vi "AdjustNames.vi"(8 "error in (no error)":errorcluster, 11 "Hardware In":T2 {"Logical Instrument"."Watchdog"."Interval (s)" min=1.0 max=360.0; "Logical Instrument"."Safety Trips"."Pmax Sink Time (s)" min=-1.0; "Logical Instrument"."Safety Trips"."Pmax Sink (W)" min=0.0 format="%#_7g"; "Logical Instrument"."Safety Trips"."Pmax Source Time (s)" min=-1.0; "Logical Instrument"."Safety Trips"."Pmax Source (W)" min=0.0 format="%#_7g"; "Logical Instrument"."Safety Trips"."Absolute Curr Peak" min=0.0; "Logical Instrument"."Safety Trips"."Imax Sink Time (s)" min=-1.0; "Logical Instrument"."Safety Trips"."Imax Sink (A)" min=0.0; "Logical Instrument"."Safety Trips"."Imax Source Time (s)" min=-1.0; "Logical Instrument"."Safety Trips"."Imax Source (A)" min=0.0; "Logical Instrument"."Safety Trips"."Absolute Volt Peak" min=0.0; "Logical Instrument"."Safety Trips"."Vmax Time (s)" min=-1.0; "Logical Instrument"."Safety Trips"."Vmax (V)" min=0.0; "Logical Instrument"."Safety Trips"."Vmin Time (s)" min=-1.0; "Logical Instrument"."Safety Trips"."Vmin (V)" min=0.0; "Logical Instrument"."Aperture (cycles)" min=1 max=64; "Logical Instrument"."FreqOut (Hz)" min=0.0 max=100.0; "Logical Instrument"."Slew Rates"."Phase Angle Min (Deg/s)" min=0.0; "Logical Instrument"."Slew Rates"."Phase Angle Max (Deg/s)" min=0.0; "Logical Instrument"."Slew Rates"."Freq Min (Hz/s)" min=0.0; "Logical Instrument"."Slew Rates"."Freq Max (Hz/s)" min=0.0; "Logical Instrument"."Slew Rates"."Pmax (W/s)" min=0.0; "Logical Instrument"."Slew Rates"."Pmin (W/s)" min=0.0; "Logical Instrument"."Slew Rates"."Imax (A/s)" min=0.0; "Logical Instrument"."Slew Rates"."Vmax (V/s)" min=0.0; "Logical Instrument"."Slew Rates"."Imin (A/s)" min=0.0; "Logical Instrument"."Slew Rates"."Vmin (V/s)" min=0.0; "Logical Instrument"."Phases"."C-Wave Shape" items=["Sine", "User1", "User2", "User3"]; "Logical Instrument"."Phases"."B-Wave Shape" items=["Sine", "User1", "User2", "User3"]; "Logical Instrument"."Phases"."A-Wave Shape" items=["Sine", "User1", "User2", "User3"]; "Logical Instrument"."Phases"."C-Change at..." min=0 max=359; "Logical Instrument"."Phases"."B-Change at..." min=0 max=359; "Logical Instrument"."Phases"."A-Change at..." min=0; "Logical Instrument"."Phases"."C-Angle (Deg)" min=0; "Logical Instrument"."Phases"."B-Angle (Deg)" min=0; "Logical Instrument"."Phases"."C-Volts (V)" min=0.0; "Logical Instrument"."Phases"."B-Volts (V)" min=0.0; "Logical Instrument"."Phases"."A-Volts (V)" min=0.0; "Logical Instrument"."Vout (V)" min=0.0; "Mode" items=["3-Phase AC"=0, "AC"=1, "DC"=2, "AC - AC"=7, "AC - DC"=8, "DC - AC"=11, "DC - DC"=12, "2-Phase AC - AC"=5, "2-Phase AC - DC"=6, "AC - AC - AC"=3, "DC - DC - DC"=4, "AC - AC - DC"=9, "AC - DC - DC"=10, "AC - DC - AC"=13, "DC - AC - AC"=14, "DC - AC - DC"=15]}) -> (0 "error out":errorcluster, 3 "Hardware Out":T2 {"Logical Instrument"."Watchdog"."Interval (s)" min=1.0 max=360.0; "Logical Instrument"."Safety Trips"."Pmax Sink Time (s)" min=-1.0; "Logical Instrument"."Safety Trips"."Pmax Sink (W)" min=0.0 format="%#_7g"; "Logical Instrument"."Safety Trips"."Pmax Source Time (s)" min=-1.0; "Logical Instrument"."Safety Trips"."Pmax Source (W)" min=0.0 format="%#_7g"; "Logical Instrument"."Safety Trips"."Absolute Curr Peak" min=0.0; "Logical Instrument"."Safety Trips"."Imax Sink Time (s)" min=-1.0; "Logical Instrument"."Safety Trips"."Imax Sink (A)" min=0.0; "Logical Instrument"."Safety Trips"."Imax Source Time (s)" min=-1.0; "Logical Instrument"."Safety Trips"."Imax Source (A)" min=0.0; "Logical Instrument"."Safety Trips"."Absolute Volt Peak" min=0.0; "Logical Instrument"."Safety Trips"."Vmax Time (s)" min=-1.0; "Logical Instrument"."Safety Trips"."Vmax (V)" min=0.0; "Logical Instrument"."Safety Trips"."Vmin Time (s)" min=-1.0; "Logical Instrument"."Safety Trips"."Vmin (V)" min=0.0; "Logical Instrument"."Aperture (cycles)" min=1 max=64; "Logical Instrument"."FreqOut (Hz)" min=0.0 max=100.0; "Logical Instrument"."Slew Rates"."Phase Angle Min (Deg/s)" min=0.0; "Logical Instrument"."Slew Rates"."Phase Angle Max (Deg/s)" min=0.0; "Logical Instrument"."Slew Rates"."Freq Min (Hz/s)" min=0.0; "Logical Instrument"."Slew Rates"."Freq Max (Hz/s)" min=0.0; "Logical Instrument"."Slew Rates"."Pmax (W/s)" min=0.0; "Logical Instrument"."Slew Rates"."Pmin (W/s)" min=0.0; "Logical Instrument"."Slew Rates"."Imax (A/s)" min=0.0; "Logical Instrument"."Slew Rates"."Vmax (V/s)" min=0.0; "Logical Instrument"."Slew Rates"."Imin (A/s)" min=0.0; "Logical Instrument"."Slew Rates"."Vmin (V/s)" min=0.0; "Logical Instrument"."Phases"."C-Wave Shape" items=["Sine", "User1", "User2", "User3"]; "Logical Instrument"."Phases"."B-Wave Shape" items=["Sine", "User1", "User2", "User3"]; "Logical Instrument"."Phases"."A-Wave Shape" items=["Sine", "User1", "User2", "User3"]; "Logical Instrument"."Phases"."C-Change at..." min=0 max=359; "Logical Instrument"."Phases"."B-Change at..." min=0 max=359; "Logical Instrument"."Phases"."A-Change at..." min=0; "Logical Instrument"."Phases"."C-Angle (Deg)" min=0; "Logical Instrument"."Phases"."B-Angle (Deg)" min=0; "Logical Instrument"."Phases"."C-Volts (V)" min=0.0; "Logical Instrument"."Phases"."B-Volts (V)" min=0.0; "Logical Instrument"."Phases"."A-Volts (V)" min=0.0; "Logical Instrument"."Vout (V)" min=0.0; "Mode" items=["3-Phase AC"=0, "AC"=1, "DC"=2, "AC - AC"=7, "AC - DC"=8, "DC - AC"=11, "DC - DC"=12, "2-Phase AC - AC"=5, "2-Phase AC - DC"=6, "AC - AC - AC"=3, "DC - DC - DC"=4, "AC - AC - DC"=9, "AC - DC - DC"=10, "AC - DC - AC"=13, "DC - AC - AC"=14, "DC - AC - DC"=15]})   [LabVIEW 2018, in "AcPwrPlugins.lvlib" / "NHRGridSim.lvclass"]
uses:
  NHRGridSim.lvclass
  TypeDefs/NHRGrid_Hardware.ctl
  TypeDefs/NHRGrid_Modes.ctl
  TypeDefs/NHRGrid_Logical_Instrument.ctl
  TypeDefs/NHRGrid_InstrumentCluster.ctl
  TypeDefs/NHRGrid_Phases_Tabs.ctl
  TypeDefs/NHRGrid_SlewRates.ctl
  TypeDefs/NHRGrid_Ranges.ctl
  TypeDefs/NHRGrid_SafetyTrips.ctl
  TypeDefs/NHRGrid_Watchdog.ctl
panel:
  in  "Tab Control":T1(tab)
  # "THIS CAN BE DELETED, WILL NOT BE USED. OLD PRELIM INTERFACE DESIGN"
  # "Degrees with Respect to Phase A"
  # "Voltages (L-N)"
  # "Degrees for Synchronization"
  # "AC Phase Waveform"
  # "Degrees with Respect to Phase A"
  # "Voltages (L-N)"
  # "Degrees for Synchronization"
  # "AC Phase Waveform"
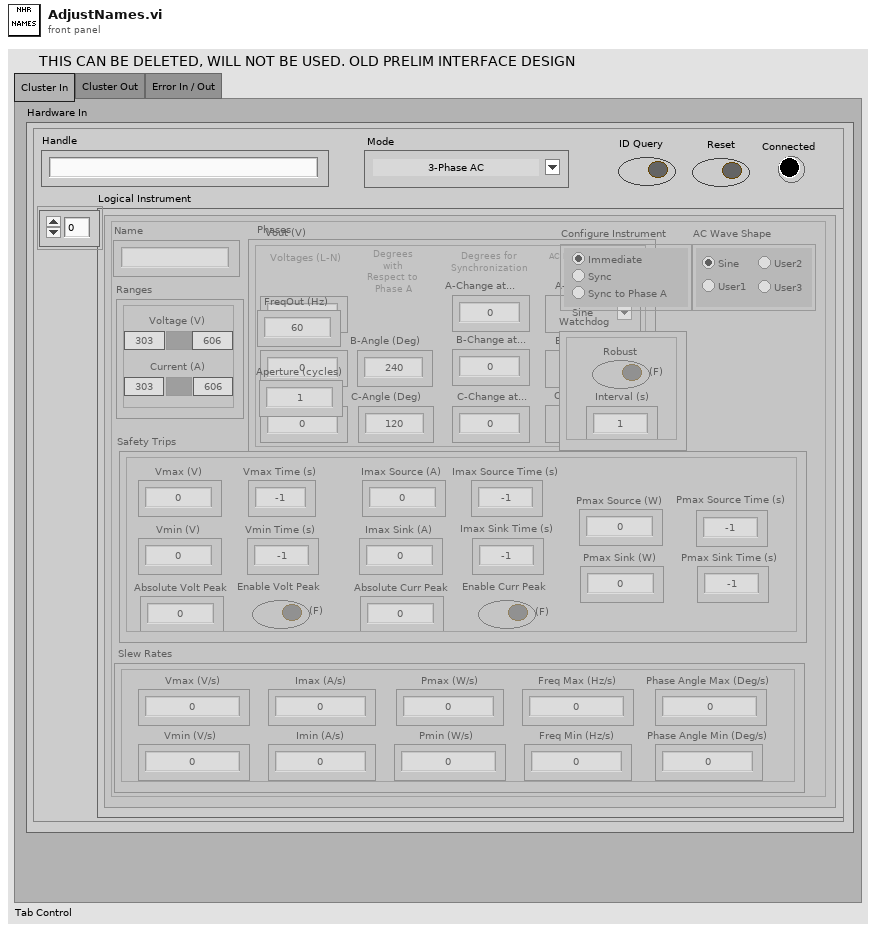
[diagram p1: front panel]
types:
  T1 = enum32{"Cluster In", "Cluster Out", "Error In / Out"}
  T2 = typedef "NHRGrid_Hardware.ctl" = cluster{"Handle":string, "Reset":bool, "Mode":T3, "ID Query":bool, "Connected":bool, "Logical Instrument":T4}
  T3 = typedef "AcPwrPlugins.lvlib/NHRGridSim.lvclass/NHRGrid_Modes.ctl" = u8
  T4 = typedef "AcPwrPlugins.lvlib/NHRGridSim.lvclass/NHRGrid_Logical_Instrument.ctl" = T5[]
  T5 = typedef "AcPwrPlugins.lvlib/NHRGridSim.lvclass/NHRGrid_InstrumentCluster.ctl" = cluster{"Name":string, "Vout (V)":dbl, "VType":string, "Phases":T6, "Slew Rates":T7, "FreqOut (Hz)":dbl, "Aperture (cycles)":i32, "Configure Instrument":enum32{"Conf1", "Conf2", "Conf3"}, "AC Wave Shape":enum32{"Sine", "User1", "User2", "User3"}, "Ranges":T8, "Safety Trips":T9, "Watchdog":T10}
  T6 = typedef "AcPwrPlugins.lvlib/NHRGridSim.lvclass/NHRGrid_Phases_Tabs.ctl" = cluster{"A-Volts (V)":dbl, "B-Volts (V)":dbl, "C-Volts (V)":dbl, "A-Change at...":i32, "B-Angle (Deg)":i32, "C-Angle (Deg)":i32, "B-Change at...":i32, "C-Change at...":i32, "AngleTxt":string, "A-Wave Shape":u16, "B-Wave Shape":u16, "C-Wave Shape":u16}
  T7 = typedef "AcPwrPlugins.lvlib/NHRGridSim.lvclass/NHRGrid_SlewRates.ctl" = cluster{"Vmax (V/s)":dbl, "Vmin (V/s)":dbl, "Imax (A/s)":dbl, "Imin (A/s)":dbl, "Pmax (W/s)":dbl, "Pmin (W/s)":dbl, "Freq Max (Hz/s)":dbl, "Freq Min (Hz/s)":dbl, "Phase Angle Max (Deg/s)":dbl, "Phase Angle Min (Deg/s)":dbl}
  T8 = typedef "AcPwrPlugins.lvlib/NHRGridSim.lvclass/NHRGrid_Ranges.ctl" = cluster{"Voltage (V)":bool, "VHi":dbl, "Current (A)":bool, "CLo":dbl, "CHi":dbl, "VLo":dbl}
  T9 = typedef "AcPwrPlugins.lvlib/NHRGridSim.lvclass/NHRGrid_SafetyTrips.ctl" = cluster{"Vmax (V)":dbl, "Vmin (V)":dbl, "Vmax Time (s)":dbl, "Vmin Time (s)":dbl, "Imax Source (A)":dbl, "Imax Sink (A)":dbl, "Imax Source Time (s)":dbl, "Imax Sink Time (s)":dbl, "Pmax Source (W)":dbl, "Pmax Sink (W)":dbl, "Pmax Source Time (s)":dbl, "Pmax Sink Time (s)":dbl, "Absolute Volt Peak":dbl, "Enable Volt Peak":bool, "Absolute Curr Peak":dbl, "Enable Curr Peak":bool, "Setting t":string, "Recomm t 2":string}
  T10 = typedef "AcPwrPlugins.lvlib/NHRGridSim.lvclass/NHRGrid_Watchdog.ctl" = cluster{"Robust":bool, "Interval (s)":dbl}
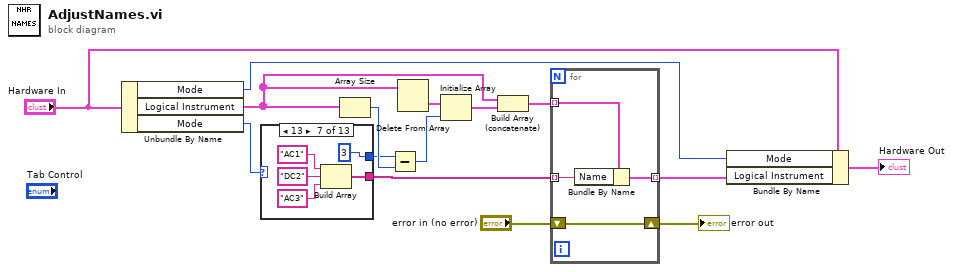
[diagram p0: block diagram]
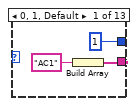
[diagram p2: hidden frame]
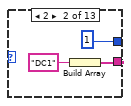
[diagram p3: hidden frame]
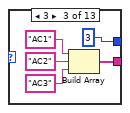
[diagram p4: hidden frame]
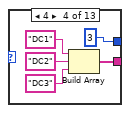
[diagram p5: hidden frame]
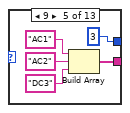
[diagram p6: hidden frame]
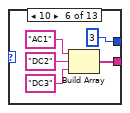
[diagram p7: hidden frame]
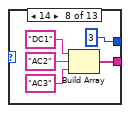
[diagram p8: hidden frame]
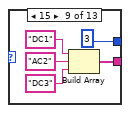
[diagram p9: hidden frame]
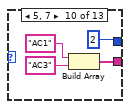
[diagram p10: hidden frame]
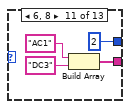
[diagram p11: hidden frame]
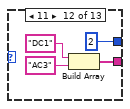
[diagram p12: hidden frame]
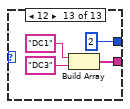
[diagram p13: hidden frame]
diagram:
  n1 = Unbundle By Name("Hardware In") -> ("Mode"=w6:T3, "Logical Instrument"=w1:T4, "Mode"=w7:T3)
  n2 = case shown="13" w7 {
    tunnel: [w17 w20 w25 w30 w35 w40 w45 w50 w55 w59 w63 w67 w71] -> w9
    tunnel: [1 1 3 3 3 3 3 3 3 2 2 2 2] -> w14
    frame 0, 1, Default {
      n3 = Build Array("AC1") -> (w17:string[])
    }
    frame 2 {
      n4 = Build Array("DC1") -> (w20:string[])
    }
    frame 3 {
      n5 = Build Array("AC1", "AC2", "AC3") -> (w25:string[])
    }
    frame 4 {
      n6 = Build Array("DC1", "DC2", "DC3") -> (w30:string[])
    }
    frame 9 {
      n7 = Build Array("AC1", "AC2", "DC3") -> (w35:string[])
    }
    frame 10 {
      n8 = Build Array("AC1", "DC2", "DC3") -> (w40:string[])
    }
    frame 13 {
      n9 = Build Array("AC1", "DC2", "AC3") -> (w45:string[])
    }
    frame 14 {
      n10 = Build Array("DC1", "AC2", "AC3") -> (w50:string[])
    }
    frame 15 {
      n11 = Build Array("DC1", "AC2", "DC3") -> (w55:string[])
    }
    frame 5, 7 {
      n12 = Build Array("AC1", "AC3") -> (w59:string[])
    }
    frame 6, 8 {
      n13 = Build Array("AC1", "DC3") -> (w63:string[])
    }
    frame 11 {
      n14 = Build Array("DC1", "AC3") -> (w67:string[])
    }
    frame 12 {
      n15 = Build Array("DC1", "DC3") -> (w71:string[])
    }
  }
  n16 = Array Size(array=w1) -> (size(s)=w15:i32)
  n17 = Subtract(x=w14, y=w15) -> (x-y=w11:i32)
  n18 = Delete From Array(array=w1) -> (deleted portion=w12:T5)  [unwired: 2 in, 1 out]
  n19 = Initialize Array(w12, w11) -> (w13:T5[])
  n20 = Build Array (concatenate)(w1, w13) -> (w10:T4)
  n21 = for {
    tunnel: w10 -> [w75] mode=indexing
    tunnel: [w74] -> w8 mode=indexing
    tunnel: w9 -> [w76] mode=indexing
    shift-right: [w73] -> w5
    shift-left: "error in (no error)" -> [w73]
    n22 = Bundle By Name(cluster=w75, "Name"=w76) -> (w74:T5)
  }
  "error out" <- w5
  n23 = Bundle By Name(cluster="Hardware In", "Mode"=w6, "Logical Instrument"=w8) -> (→"Hardware Out":T2)
